vi "valve VCH check.vi"() -> ()   [LabVIEW 2019]
uses:
  ctl/Z_State_VCH.ctl
  ctl/Zr_control_VCH.ctl
  ctl/Zr_control_short_VCH.ctl
  ctl/Z_control_VCH.ctl
  ctl/Z_short.ctl
  c6493a95-7405-460f-ab8c-2c96f87d346a.vi
  <vilib>/JDP Science/JSONtext/Find Multiple Items.vi
  <vilib>/JDP Science/JSONtext/String Subset.vi
  <vilib>/JDP Science/JSONtext/support/Strip Quotes and Unescape.vi
  <vilib>/JDP Science/JSONtext/JSON text to Variant.vi
  <vilib>/JDP Science/JSONtext/Parsing/Parse Full Path or Item Name.vi
  <vilib>/JDP Science/JSONtext/Offset/Find Item Locations by Path.vi
  <vilib>/JDP Science/JSONtext/support/Unescape JSON string.vi
  Valves.lvlib
  OPC/OPC addons.lvlib
panel:
  in  "Z_ASetState":T1=enum."closed ready"
  out "JSON string":string
  in  "View visu":bool
  in  "Parameters table VCH":u32[](array[numeric])=[0, 10000, 0, 0, 100, 100, 0, 3000, 1000, 100, 3]
  in  "ALR":cluster{"ALRL1":bool, "ALRL2":bool}
  out "Y":bool[](array[boolean])
  out "ALR_ON":bool[](array[boolean])
  out "This VI":refnum<vi>
  out "reset out":bool
  # "T_valve_open_state"
  # "T_restart_delay"
  # "T_valve_open"
  # "T_valve_close"
  # "T_little_pause"
  # "T_start_delay"
  # "T_stop_delay"
  # "T_big_pause"
  # "N_repeat"
  # "T_check"
  # "TsStop"
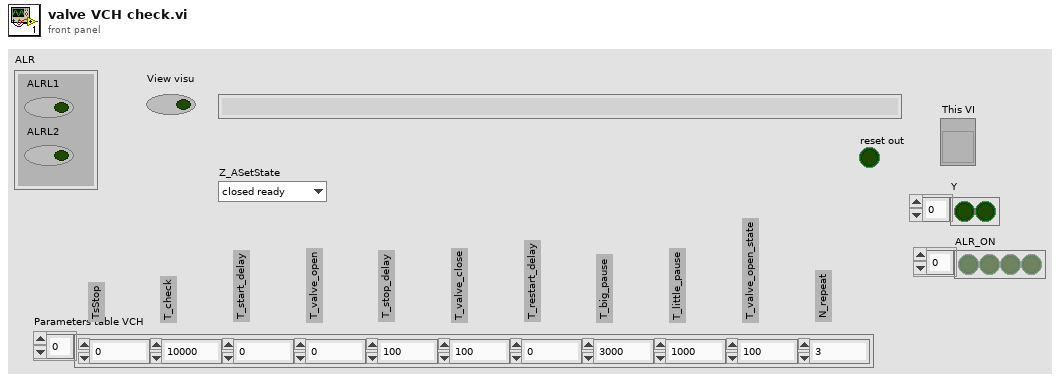
[diagram p1: front panel]
types:
  T1 = typedef "Valves.lvlib/Z_State_VCH.ctl" = enum8{"initialization", "alarm", "disabled", "not ready", "closed ready", "reserv", "reserv1", "reserv2", "reserv3", "check", "on min", "open", "on (closed)"}
  T2 = typedef "Valves.lvlib/Z_short.ctl" = cluster{"Z_Source":u8, "Z_SetState":u8, "Z_State":u8, "Z_State_T":u32, "ZM_State":u8, "ZM_State_T":u32, "ALR  L1":bool, "ALR  L2":bool, "HH_run":i32}
  T3 = typedef "Valves.lvlib/Z_control_VCH.ctl" = cluster{"Z_HSw":u8, "Z_HSetState":T1, "Z_ASetState":T1, "Z_DSetState":T1}
  T4 = typedef "Valves.lvlib/Zr_control_short_VCH.ctl" = cluster{"Z_HSw":u8, "Z_HSetState":u8, "Reset_ALR":bool}
  T5 = typedef "Valves.lvlib/Zr_control_VCH.ctl" = cluster{"Z_HSw":u8, "Z_HSetState":T1, "Reset_ALR":bool}
  T6 = typedef "Valves.lvlib/Z.ctl" = cluster{"Z_Source":T7, "Z_SetState":T1, "Z_State":T1, "Z_State_T":u32, "ZM_State":T8, "ZM_State_T":u32, "ALR  L1":bool, "ALR  L2":bool, "HH_run":i32}
  T7 = typedef "Heating.lvlib/Y_source.ctl" = enum8{"initialize", "local disabled", "local hand", "hand", "auto", "dist"}
  T8 = typedef "Valves.lvlib/ZM_State_VCH.ctl" = enum8{"initialization", "closed", "big_pause", "little_pause", "open", "close_cmd"}
  T9 = enum32{"Invalid", "Standard", "Closed", "Hidden", "Minimized", "Maximized"}
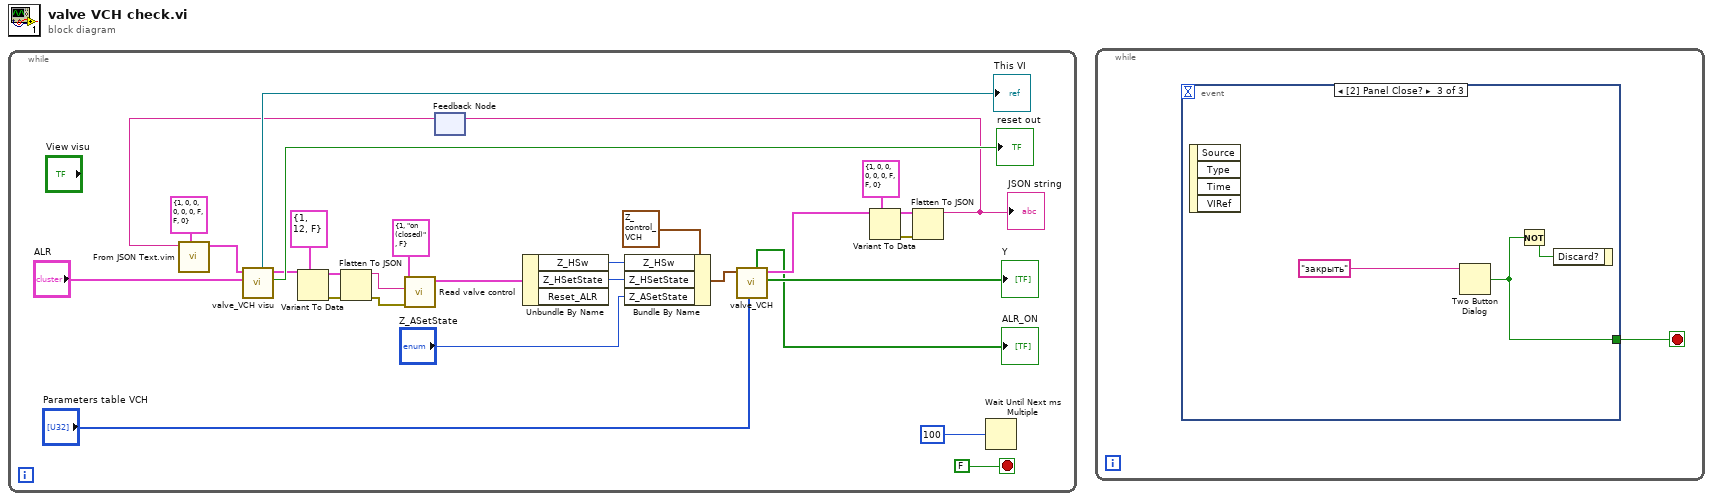
[diagram p0: block diagram]
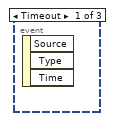
[diagram p2: hidden frame]
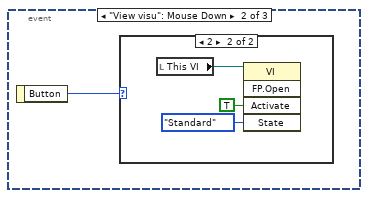
[diagram p3: hidden frame]
diagram:
  n1 = while {
    stop <- FALSE stop-if-true
    n2 = feedback #1() -> (w19:string)  [unwired: 1 in]
    n3 = call "From JSON Text.vim"("Data Type and Default Value"=T2 {"Z_Source"=1, "Z_SetState"=0, "Z_State"=0, "Z_State_T"=0, "ZM_State"=0, "ZM_State_T"=0, "ALR  L1"=FALSE, "ALR  L2"=FALSE, "HH_run"=0} ("Z"), "JSON"=w19) -> ("Data out"=w20:T2)  [unwired: 8 in, 1 out]
    n4 = call "valve_VCH visu.vi"("ALR"="ALR", "Z"=w20) -> ("reset out"=→"reset out":bool, "Z_SetState"=w16:T5, "This VI"=→"This VI":refnum<vi>)  [unwired: 7 in]
    n5 = Variant To Data(type=T4 {"Z_HSw"=1, "Z_HSetState"=12, "Reset_ALR"=FALSE} ("HT_in in"), Variant=w16) -> (data=w14:T4, error out=w17:errorcluster)  [unwired: 1 in]
    n6 = Flatten To JSON(anything=w14, error in (no error)=w17) -> (JSON string=w13:string, 11:w12:errorcluster)  [unwired: 1 in]
    n7 = call "Read valve control.vi"("error in (no error)"=w12, "value"=w13, "HT_in in"=T5 {"Z_HSw"=1, "Z_HSetState"=enum."on (closed)", "Reset_ALR"=FALSE}) -> ("HT1_in out"=w21:T5)  [unwired: 6 in, 2 out]
    n8 = Unbundle By Name(w21) -> ("Z_HSw"=w8:u8, "Z_HSetState"=w7:T1)  [unwired: 1 out]
    n9 = Bundle By Name(cluster=T3 {"Z_HSw"=1, "Z_HSetState"=enum."on (closed)", "Z_ASetState"=enum."closed ready", "Z_DSetState"=enum."closed ready"} ("Z_control"), "Z_HSw"=w8, "Z_HSetState"=w7, "Z_ASetState"="Z_ASetState") -> (w9:T3)
    n10 = call "valve_VCH.vi"("Parameters table VCH"="Parameters table VCH", "Z_control"=w9) -> ("YB"=→"Y":bool[], "Z_State"=w22:T6, "ALR_ON"=→"ALR_ON":bool[])  [unwired: 6 in, 1 out]
    n11 = Variant To Data(type=T2 {"Z_Source"=1, "Z_SetState"=0, "Z_State"=0, "Z_State_T"=0, "ZM_State"=0, "ZM_State_T"=0, "ALR  L1"=FALSE, "ALR  L2"=FALSE, "HH_run"=0} ("Z"), Variant=w22) -> (data=w5:T2, error out=w4:errorcluster)  [unwired: 1 in]
    n12 = Flatten To JSON(anything=w5, error in (no error)=w4) -> (JSON string=w3:string)  [unwired: 1 in, 1 out]
    "JSON string" <- w3
    n13 = feedback-in #1(w3) -> ()
    n14 = Wait Until Next ms Multiple(millisecond multiple=u32 100) -> ()  [unwired: 1 out]
  }
  n15 = while {
    stop <- w30 stop-if-true
    n16 = event shown="[2] Panel Close?" {
      selector: _ -> [_ _ _]
      dyn-events: _ -> [_ _ _]
      timeout: _ -> [_ _ _]
      tunnel: [_ _ w36] -> w30
      event Timeout {
        n17 = event-data() -> ()  [unwired: 1 in, 3 out]
      }
      event "View visu": Mouse Down {
        n18 = event-data() -> ("Button"=w31:u16)  [unwired: 1 in]
        n19 = case shown="2" w31 {
          frame 0, Default {
          }
          frame 2 {
            n20 = local read "This VI"() -> (w34:refnum<vi>)
            n21 = invoke class="VI" method="FP.Open"(reference=w34, "Activate"=TRUE ("Activate?"), "State"=T9."Standard") -> ()  [unwired: 2 in, 5 out]
          }
        }
      }
      event Panel Close? {
        n22 = event-data() -> ()  [unwired: 1 in, 4 out]
        n23 = Two Button Dialog(message="закрыть") -> (T button?=w36:bool)  [unwired: 2 in]
        n24 = Not(x=w36) -> (.not. x?=w35:bool)
        n25 = event-data("Discard?"=w35) -> ()  [unwired: 1 in, 1 out]
      }
    }
  }
